vi "Test Result File Name Global.vi"() -> ()   [LabVIEW 2018]
panel:
  in  "Results Parent Dir":path=path "C:/RageATE Results"
  out "Test Results File Name":path
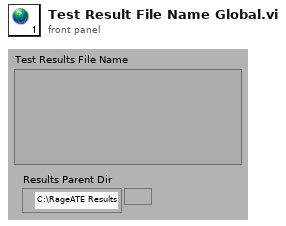
[diagram p1: front panel]
diagram:
